vi "ODrive velocity control and error managment.vi"(8 "error in (no error)":errorcluster, 11 "Refnum in":refnum<k20>) -> (0 "Error out":errorcluster, 3 "Refnum out":refnum<k20>)   [LabVIEW 2016]
uses:
  Typedef/Remote Control Cluster.ctl
  Shared resoruces/Front Panel Control Variables.vi
  <vilib>/Utility/error.llb/Error Cluster From Error Code.vi
  <vilib>/rvi/errors/niLvFpgaAdjustHostInterfaceError.vi
  <vilib>/RVI Host/nirviSupport.llb/nirviErrorClusterFromErrorCode.vi
  <vilib>/rvi/interface/nirviMethod/nirviMethod.xnode
  <vilib>/rvi/interface/nirviReadWriteControl/nirviReadWriteControl.xnode
  <vilib>/FPGAPlugInAG/Dynamic/niLvFpga_WriteFifo_Dynamic.vi
  <vilib>/rvi/errors/niLvFpgaMergeErrorWithErrorCode.vi
  Shared resoruces/Shared resources RT.lvlib
  NiFpgaLv.dll
  <vilib>/rvi/interface/Simulation/niFpgaSimulationCallBeginRW.vi
  <vilib>/rvi/interface/nirviMethod/StockFPGA_InlinedMethodWaitForSingleIRQ.vi
  <vilib>/FPGAPlugInAG/Dynamic/niLvFpga_WaitOnIrq_Dynamic.vi
  <vilib>/FPGAPlugInAG/Dynamic/niLvFpga_AcknowledgeIrq_Dynamic.vi
panel:
  in  "maxDiff":i16=5
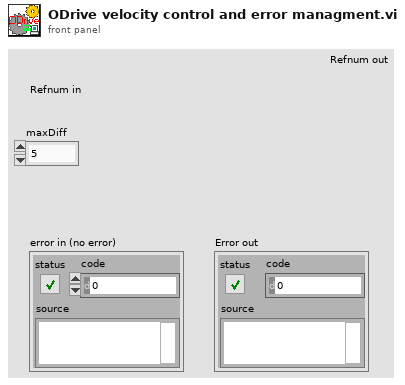
[diagram p1: front panel]
types:
  T1 = typedef "Remote Control Cluster.ctl" = cluster{"Pot1":u16, "Pot2":u16, "Pot3":u16, "Pot4":u16, "Switch1":cluster{"L":bool, "H":bool}, "Switch2":cluster{"L":bool, "H":bool}, "Switch3":cluster{"L":bool, "H":bool}}
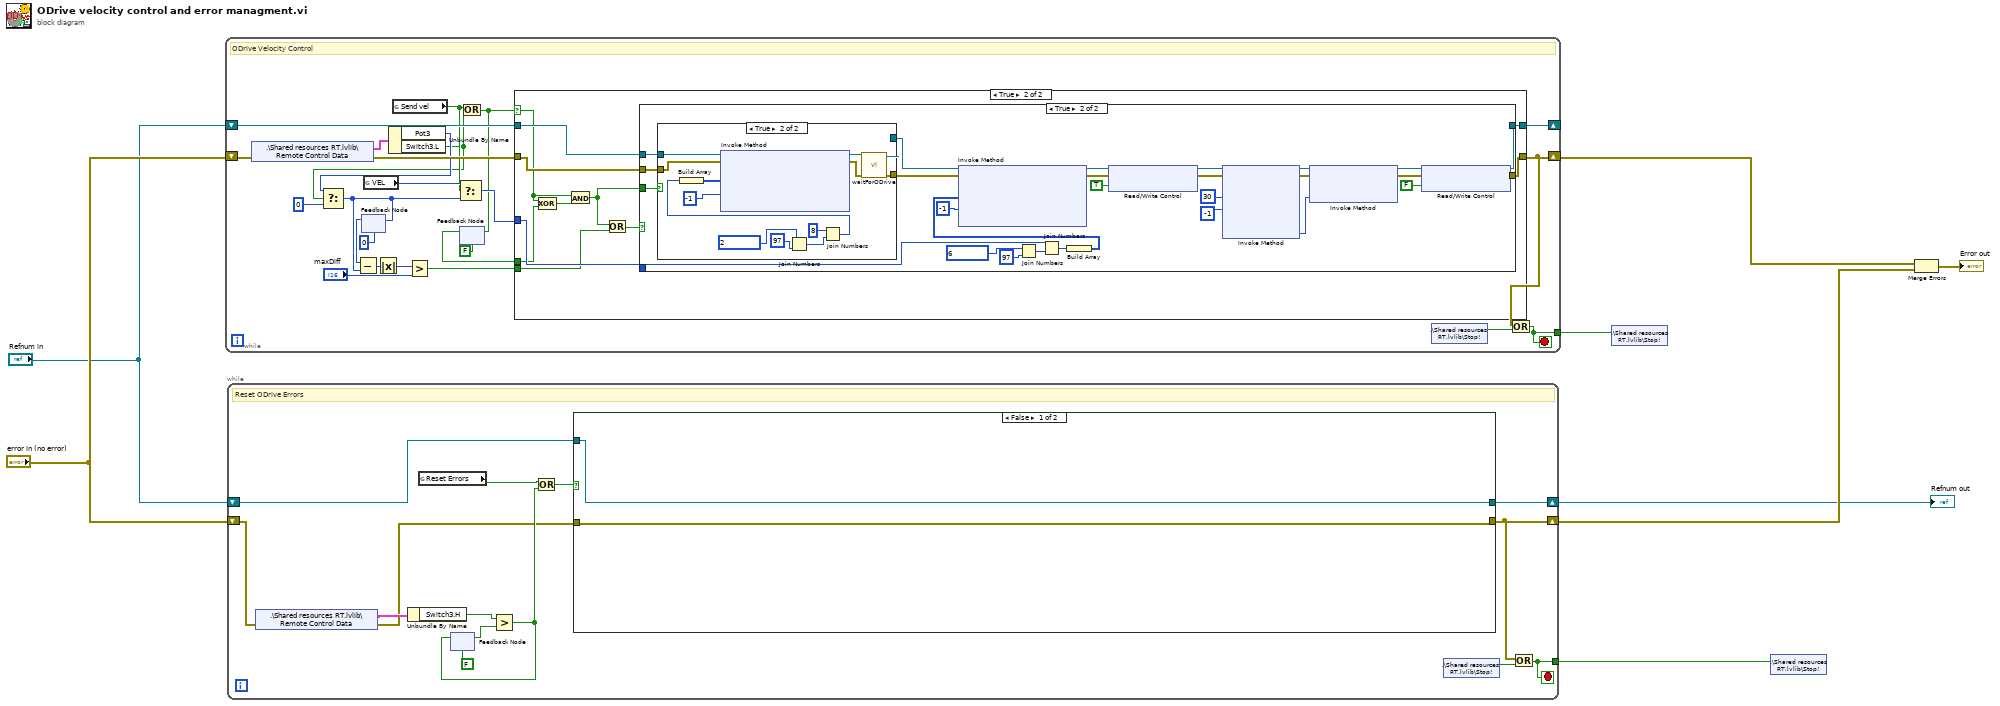
[diagram p0: block diagram]
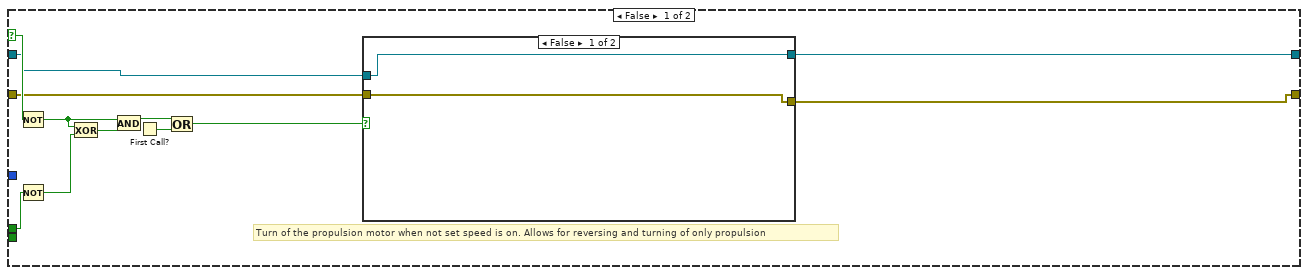
[diagram p2: hidden frame]
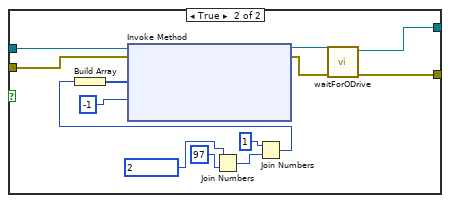
[diagram p3: hidden frame]
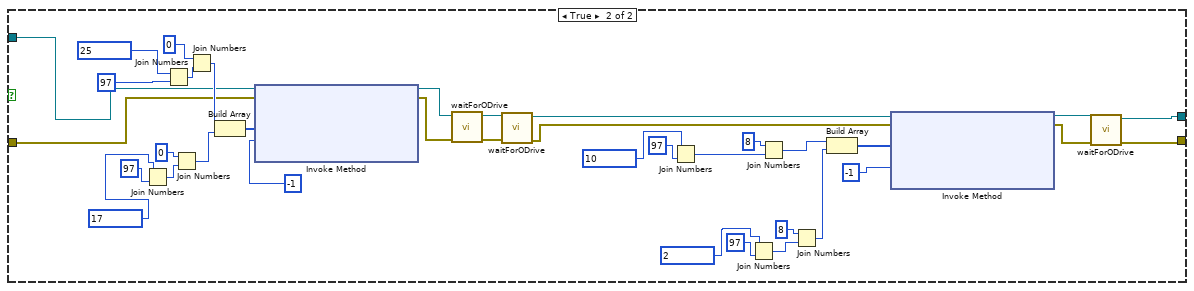
[diagram p6: hidden frame]
diagram:
  n1 = while {
    shift-right: [w32] -> _
    shift-left: "Refnum in" -> [w31]
    shift-right: [w26] -> w3
    shift-left: "error in (no error)" -> [w30]
    tunnel: [w25] -> w6
    stop <- w25 stop-if-true
    # "ODrive Velocity Control"
    n2 = shared-variable ".\\Shared resources RT.lvlib\\Remote Control Data"(error in=w30) -> (w28:T1, error out=w29:errorcluster)
    n3 = feedback #1(u16 0) -> (w20:u16)
    n4 = global read "Front Panel Control Variables.vi" "VEL"() -> (w23:u16)
    n5 = Unbundle By Name(w28) -> ("Pot3"=w14:u16, "Switch3.L"=w13:bool)
    n6 = Select(t=w14, s=w13, f=u16 0) -> (s? t:f=w15:u16)
    n7 = Subtract(x=w20, y=w15) -> (x-y=w19:i16)
    n8 = feedback-in #1(w15) -> ()
    n9 = Absolute Value(x=w19) -> (abs(x)=w18:i16)
    n10 = global read "Front Panel Control Variables.vi" "Send vel"() -> (w22:bool)
    n11 = Greater?(x=w18, y="maxDiff") -> (0:w10:bool)
    n12 = Select(t=w23, s=w22, f=w15) -> (s? t:f=w24:u16)
    n13 = Or(x=w22, y=w13) -> (x .or. y?=w9:bool)
    n14 = feedback-in #2(w9) -> ()
    n15 = feedback #2(FALSE) -> (w11:bool)
    n16 = case shown="True" w9 {
      selector: w9 -> [w42 w64]
      tunnel: w24 -> [_ w70]
      tunnel: [w39 w69] -> w26
      tunnel: [w38 w68] -> w32
      tunnel: w29 -> [w40 w67]
      tunnel: w31 -> [w41 w66]
      tunnel: w11 -> [w33 w63]
      tunnel: w10 -> [_ w62]
      frame False {
        # "Turn of the propulsion motor when not set speed is on. Allows for reversing and turning of only propulsion"
        n17 = Not(x=w42) -> (.not. x?=w43:bool)
        n18 = Not(x=w33) -> (.not. x?=w36:bool)
        n19 = Exclusive Or(1:w36, 2:w43) -> (0:w44:bool)
        n20 = And(x=w43, y=w44) -> (x .and. y?=w37:bool)
        n21 = First Call?() -> (First Call?: T/F=w34:bool)
        n22 = Or(x=w37, y=w34) -> (x .or. y?=w35:bool)
        n23 = case shown="False" w35 {
          tunnel: w41 -> [w45 w50]
          tunnel: w40 -> [w46 w49]
          tunnel: [w46 w48] -> w39
          tunnel: [w45 w47] -> w38
          frame False {
          }
          frame True {
            n24 = Join Numbers(hi=u8 2 ("lo"), lo=u8 97) -> ((hi.lo)=w57:u16)
            n25 = Join Numbers(hi=u16 1, lo=w57) -> ((hi.lo)=w54:u32)
            n26 = Build Array(w54) -> (w59:u32[])
            n27 = xnode "Invoke Method"("FPGA VI Reference In"=w50, "error in"=w49, "Data"=w59, "Timeout (ms)"=-1) -> ("FPGA VI Reference Out"=w52:refnum<k20>, "error out"=w51:errorcluster)  [unwired: 1 out]
            n28 = call "waitForODrive.vi"("error in (no error)"=w51, "Refnum in"=w52) -> ("error out"=w48:errorcluster, "Refnum out"=w47:refnum<k20>)  [unwired: 8 in]
          }
        }
      }
      frame True {
        n29 = Exclusive Or(1:w63, 2:w64) -> (0:w65:bool)
        n30 = And(x=w64, y=w65) -> (x .and. y?=w60:bool)
        n31 = Or(x=w60, y=w62) -> (x .or. y?=w61:bool)
        n32 = case shown="True" w61 {
          tunnel: w70 -> [_ w80]
          tunnel: [w72 w79] -> w69
          tunnel: [w71 w78] -> w68
          tunnel: w67 -> [w72 w76]
          tunnel: w66 -> [w71 w75]
          tunnel: w60 -> [_ w73]
          frame False {
          }
          frame True {
            n33 = case shown="True" w73 {
              tunnel: w75 -> [w100 w105]
              tunnel: w76 -> [w101 w104]
              tunnel: [w101 w103] -> w77
              tunnel: [w100 w102] -> w74
              frame False {
              }
              frame True {
                n34 = Join Numbers(hi=u8 2 ("lo"), lo=u8 97) -> ((hi.lo)=w112:u16)
                n35 = Join Numbers(hi=u16 8, lo=w112) -> ((hi.lo)=w109:u32)
                n36 = Build Array(w109) -> (w114:u32[])
                n37 = xnode "Invoke Method"("FPGA VI Reference In"=w105, "error in"=w104, "Data"=w114, "Timeout (ms)"=-1) -> ("FPGA VI Reference Out"=w107:refnum<k20>, "error out"=w106:errorcluster)  [unwired: 1 out]
                n38 = call "waitForODrive.vi"("error in (no error)"=w106, "Refnum in"=w107) -> ("error out"=w103:errorcluster, "Refnum out"=w102:refnum<k20>)  [unwired: 8 in]
              }
            }
            n39 = Join Numbers(hi=u8 6 ("lo"), lo=u8 97) -> ((hi.lo)=w84:u16)
            n40 = Join Numbers(hi=w80, lo=w84) -> ((hi.lo)=w83:u32)
            n41 = Build Array(w83) -> (w81:u32[])
            n42 = xnode "Invoke Method"("FPGA VI Reference In"=w74, "error in"=w77, "Data"=w81, "Timeout (ms)"=-1) -> ("FPGA VI Reference Out"=w88:refnum<k20>, "error out"=w89:errorcluster)  [unwired: 1 out]
            n43 = xnode "Read/Write Control"("FPGA VI Reference In"=w88, "error in"=w89, "ODrive RT Control"=TRUE) -> ("FPGA VI Reference Out"=w87:refnum<k20>, "error out"=w86:errorcluster)
            n44 = xnode "Invoke Method"("FPGA VI Reference In"=w87, "error in"=w86, "IRQ Number(s)"=30, "Timeout (ms)"=-1) -> ("FPGA VI Reference Out"=w98:refnum<k20>, "error out"=w95:errorcluster, "IRQ(s) Asserted"=w96:i32)  [unwired: 1 out]
            n45 = xnode "Invoke Method"("FPGA VI Reference In"=w98, "error in"=w95, "IRQ Number(s)"=w96) -> ("FPGA VI Reference Out"=w93:refnum<k20>, "error out"=w92:errorcluster)
            n46 = xnode "Read/Write Control"("FPGA VI Reference In"=w93, "error in"=w92, "ODrive RT Control"=FALSE) -> ("FPGA VI Reference Out"=w78:refnum<k20>, "error out"=w79:errorcluster)
          }
        }
      }
    }
    n47 = shared-variable ".\\Shared resources RT.lvlib\\Stop!"() -> (w27:bool)  [unwired: 1 in, 1 out]
    n48 = Or(x=w26, y=w27) -> (x .or. y?=w25:bool)
  }
  n49 = while {
    shift-right: [w127] -> w1
    shift-left: "Refnum in" -> [w128]
    shift-right: [w117] -> w4
    shift-left: "error in (no error)" -> [w119]
    tunnel: [w116] -> w5
    stop <- w116 stop-if-true
    # "Reset ODrive Errors"
    n50 = shared-variable ".\\Shared resources RT.lvlib\\Remote Control Data"(error in=w119) -> (w121:T1, error out=w120:errorcluster)
    n51 = Unbundle By Name(w121) -> ("Switch3.H"=w126:bool)
    n52 = global read "Front Panel Control Variables.vi" "Reset Errors"() -> (w115:bool)
    n53 = feedback #3(FALSE) -> (w125:bool)
    n54 = Greater?(x=w126, y=w125) -> (0:w123:bool)
    n55 = feedback-in #3(w123) -> ()
    n56 = Or(x=w115, y=w123) -> (x .or. y?=w122:bool)
    n57 = case shown="False" w122 {
      tunnel: w128 -> [w130 w150]
      tunnel: w120 -> [w129 w149]
      tunnel: [w130 w132] -> w127
      tunnel: [w129 w131] -> w117
      frame False {
      }
      frame True {
        n58 = Join Numbers(hi=u8 17 ("lo"), lo=u8 97) -> ((hi.lo)=w155:u16)
        n59 = Join Numbers(hi=u8 25 ("lo"), lo=u8 97) -> ((hi.lo)=w166:u16)
        n60 = Join Numbers(hi=u16 0, lo=w155) -> ((hi.lo)=w153:u32)
        n61 = Join Numbers(hi=u16 0, lo=w166) -> ((hi.lo)=w164:u32)
        n62 = Build Array(w164, w153) -> (w163:u32[])
        n63 = xnode "Invoke Method"("FPGA VI Reference In"=w150, "error in"=w149, "Data"=w163, "Timeout (ms)"=-1) -> ("FPGA VI Reference Out"=w160:refnum<k20>, "error out"=w161:errorcluster)  [unwired: 1 out]
        n64 = call "waitForODrive.vi"("error in (no error)"=w161, "Refnum in"=w160) -> ("error out"=w152:errorcluster, "Refnum out"=w151:refnum<k20>)  [unwired: 8 in]
        n65 = call "waitForODrive.vi"("error in (no error)"=w152, "Refnum in"=w151) -> ("error out"=w135:errorcluster, "Refnum out"=w136:refnum<k20>)  [unwired: 8 in]
        n66 = Join Numbers(hi=u8 10 ("lo"), lo=u8 97) -> ((hi.lo)=w145:u16)
        n67 = Join Numbers(hi=u8 2 ("lo"), lo=u8 97) -> ((hi.lo)=w141:u16)
        n68 = Join Numbers(hi=u16 8, lo=w145) -> ((hi.lo)=w147:u32)
        n69 = Join Numbers(hi=u16 8, lo=w141) -> ((hi.lo)=w138:u32)
        n70 = Build Array(w147, w138) -> (w148:u32[])
        n71 = xnode "Invoke Method"("FPGA VI Reference In"=w136, "error in"=w135, "Data"=w148, "Timeout (ms)"=-1) -> ("FPGA VI Reference Out"=w134:refnum<k20>, "error out"=w133:errorcluster)  [unwired: 1 out]
        n72 = call "waitForODrive.vi"("error in (no error)"=w133, "Refnum in"=w134) -> ("error out"=w131:errorcluster, "Refnum out"=w132:refnum<k20>)  [unwired: 8 in]
      }
    }
    n73 = shared-variable ".\\Shared resources RT.lvlib\\Stop!"() -> (w118:bool)  [unwired: 1 in, 1 out]
    n74 = Or(x=w117, y=w118) -> (x .or. y?=w116:bool)
  }
  "Refnum out" <- w1
  n75 = shared-variable ".\\Shared resources RT.lvlib\\Stop!"(w6) -> ()  [unwired: 1 in, 1 out]
  n76 = shared-variable ".\\Shared resources RT.lvlib\\Stop!"(w5) -> ()  [unwired: 1 in, 1 out]
  n77 = Merge Errors(w3, w4) -> (→"Error out":errorcluster)
